vi "QPMX Open.vi"(8 "error in":errorcluster, 11 "QPMX ssn":T1={"visa"="", "switch mode"=enum."Switched by TWM", "sequence"=[], "timing delays"=[], "polarity"=enum."Positive", "ss delay (s)"=2.0, "internal timer (s)"=1.0, "Last loaded sequence file"=path "", "startup delay (s)"=2000.0} {"startup delay (s)" min=0.0 step=1.0; "internal timer (s)" min=0.0 step=1.0; "ss delay (s)" min=0.0 step=1.0; "timing delays" min=1 max=255 step=1}) -> (0 "error out":errorcluster, 2 "idn string":string, 3 "QPMX ssn out":T1={"visa"="", "switch mode"=enum."Switched by TWM", "sequence"=[], "timing delays"=[], "polarity"=enum."Positive", "ss delay (s)"=2.0, "internal timer (s)"=1.0, "Last loaded sequence file"=path "", "startup delay (s)"=2000.0} {"startup delay (s)" min=0.0 step=1.0; "internal timer (s)" min=0.0 step=1.0; "ss delay (s)" min=0.0 step=1.0; "timing delays" min=1 max=255 step=1})   [LabVIEW 2020]
doc: "Wrapper layer between TWM and QuPMXdriver. Initialize multiplexer."
uses:
  Generic COM/QPMX Session.ctl
  QPMX switch mode.ctl
  QPMX polarity.ctl
  QuPMXLabVIEWdriver/QuPMXdriver.lvlib
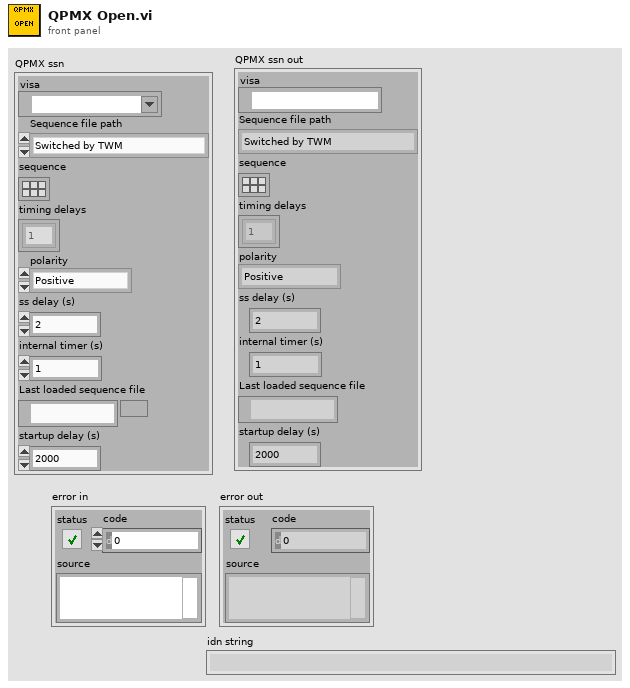
[diagram p1: front panel]
types:
  T1 = typedef "QPMX Session.ctl" = cluster{"visa":refnum<visa-resource-name>, "switch mode":T2, "sequence":bool[][], "timing delays":u32[], "polarity":T3, "ss delay (s)":dbl, "internal timer (s)":dbl, "Last loaded sequence file":path, "startup delay (s)":dbl}
  T2 = typedef "QPMX switch mode.ctl" = enum16{"Switched by TWM", "Switched by external clock", "Switched by internal clock"}
  T3 = typedef "QPMX polarity.ctl" = enum16{"Positive", "Negative"}
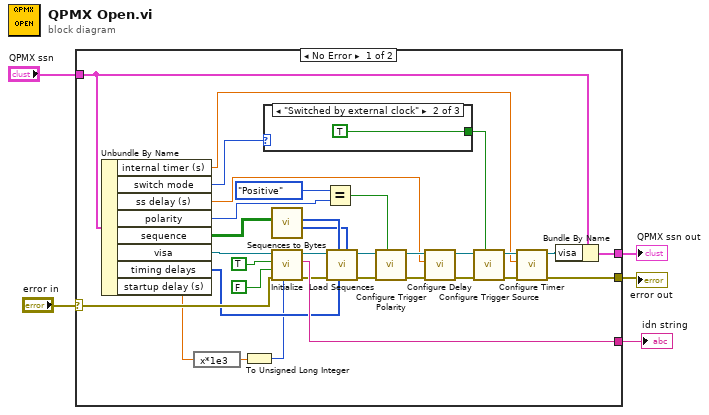
[diagram p0: block diagram]
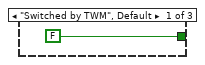
[diagram p2: hidden frame]
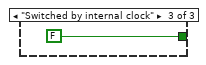
[diagram p3: hidden frame]
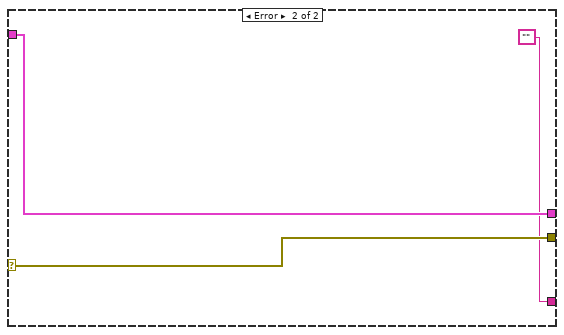
[diagram p4: hidden frame]
diagram:
  n1 = case shown="No Error" "error in" {
    selector: "error in" -> [w38 w44]
    tunnel: [w12 w44] -> w3
    tunnel: [w32 ""] -> w4
    tunnel: "QPMX ssn" -> [w34 w43]
    tunnel: [w33 w43] -> w1
    frame No Error {
      n2 = Unbundle By Name(w34) -> ("internal timer (s)"=w9:dbl, "switch mode"=w15:T2, "ss delay (s)"=w18:dbl, "polarity"=w19:T3, "sequence"=w20:bool[][], "visa"=w37:refnum<visa-resource-name>, "timing delays"=w29:u32[], "startup delay (s)"=w7:dbl)
      n3 = expression code="x*1e3"(w7) -> (w8:dbl)
      n4 = To Unsigned Long Integer(number=w8) -> (unsigned 32bit integer=w6:u32)
      n5 = case shown="\"Switched by external clock\"" w15 {
        tunnel: [FALSE ("Trigger External (T)") TRUE ("Trigger External (T)") FALSE ("Trigger External (T)")] -> w14
        frame "Switched by TWM", Default {
        }
        frame "Switched by external clock" {
        }
        frame "Switched by internal clock" {
        }
      }
      n6 = call "Sequences to Bytes.vi"("Channel states"=w20) -> ("Ch. bytes 2"=w30:u8[], "Ch. bytes 1"=w31:u8[])  [unwired: 9 in]
      n7 = call "Initialize.vi"("Startup delay (0 ms)"=w6, "error in (no error)"=w38, "Reset (False)"=FALSE ("Reset (True)"), "ID Query (True)"=TRUE, "VISA resource name"=w37) -> ("error out"=w28:errorcluster, "ID"=w32:string, "VISA resource name out"=w27:refnum<visa-resource-name>)  [unwired: 4 in]
      n8 = Equal?(x=QPMX_polarity."Positive" ("y"), y=w19) -> (x = y?=w21:bool)
      n9 = call "Load Sequences.vi"("Byte 2 Ch."=w30, "Byte 3 Timing Delay"=w29, "Byte 1 Ch."=w31, "error in (no error)"=w28, "VISA resource name"=w27) -> ("error out"=w25:errorcluster, "VISA resource name out"=w26:refnum<visa-resource-name>)  [unwired: 5 in]
      n10 = call "Configure Trigger Polarity.vi"("Trigger Polarity Positive (T)"=w21, "error in (no error)"=w25, "VISA resource name"=w26) -> ("error out"=w24:errorcluster, "VISA resource name out"=w23:refnum<visa-resource-name>)  [unwired: 7 in]
      n11 = call "Configure Delay.vi"("error in (no error)"=w24, "Delay (s)"=w18, "VISA resource name"=w23) -> ("error out"=w17:errorcluster, "VISA resource name out"=w16:refnum<visa-resource-name>)  [unwired: 7 in]
      n12 = call "Configure Trigger Source.vi"("Trigger External (T)"=w14, "error in (no error)"=w17, "VISA resource name"=w16) -> ("error out"=w13:errorcluster, "VISA resource name out"=w10:refnum<visa-resource-name>)  [unwired: 7 in]
      n13 = call "Configure Timer.vi"("error in (no error)"=w13, "Internal timer (2 s)"=w9, "VISA resource name"=w10) -> ("error out"=w12:errorcluster, "VISA resource name out"=w11:refnum<visa-resource-name>)  [unwired: 7 in]
      n14 = Bundle By Name(cluster=w34, "visa"=w11) -> (w33:T1)
    }
    frame Error {
    }
  }
  "error out" <- w3
  "idn string" <- w4
  "QPMX ssn out" <- w1
